vi "RandomNumberWithinRange.vi"(1 "High":i32, 4 "Low":i32) -> (22 "Random Number":i32)   [LabVIEW 2015]
doc: "Generates a random number between High and Low inputs."
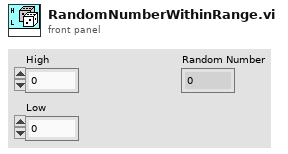
[diagram p1: front panel]
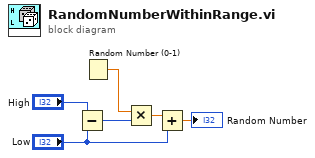
[diagram p0: block diagram]
diagram:
  n1 = Subtract(x="High", y="Low") -> (x-y=w4:i32)
  n2 = Random Number (0-1)() -> (number: 0 to 1=w1:dbl)
  n3 = Multiply(x=w1, y=w4) -> (x*y=w6:dbl)
  n4 = Add(x=w6, y="Low") -> (x+y=→"Random Number":dbl)
